vi "Write daemon error.vi"(8 "error in (no error)":errorcluster, 10 "daemon error":errorcluster, 11 "Network Slave in":refnum<class "WebSocket Server.lvclass">) -> (0 "error out":errorcluster, 3 "Network Slave out":refnum<class "WebSocket Server.lvclass">)   [LabVIEW 2021, in "WebSockets.lvlib" / "WebSocket Server.lvclass"]
uses:
  WebSocket Server.lvclass
  WebSocket Server.lvclass/WebSocket Server.ctl
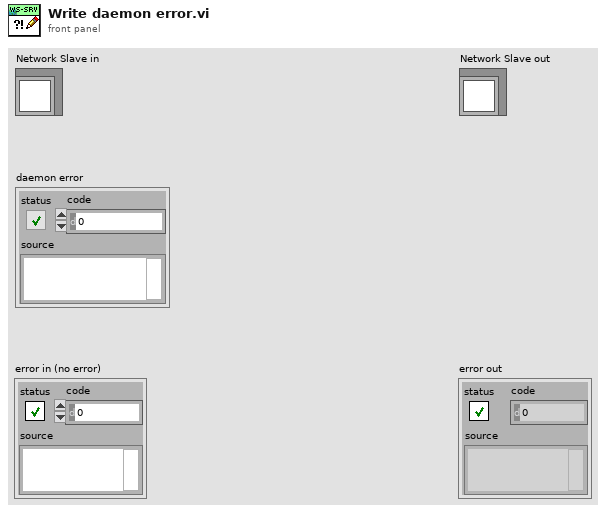
[diagram p1: front panel]
types:
  T1 = typedef "WebSockets.lvlib/WebSocket Server.lvclass/daemon status cluster.ctl" = cluster{"error":errorcluster, "status":T2}
  T2 = typedef "WebSockets.lvlib/WebSocket Server.lvclass/daemon status.ctl" = enum16{"Not Started", "Running", "Error", "Stopped"}
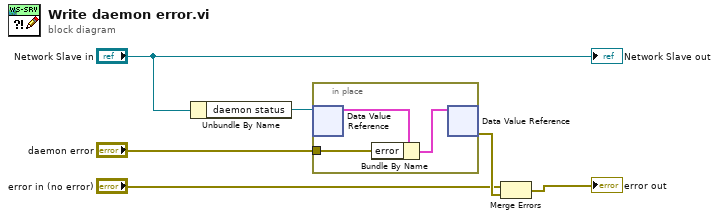
[diagram p0: block diagram]
diagram:
  n1 = Unbundle By Name("Network Slave in") -> ("daemon status"=w5:refnum<data-value>)
  n2 = in-place {
    in-place-border: "daemon error" -> [w7]
    n3 = in-place-dvr #1(w5) -> (w9:T1)  [unwired: 1 out]
    n4 = Bundle By Name(cluster=w9, "error"=w7) -> (w8:T1)
    n5 = in-place-dvr #1(w8) -> (w6:errorcluster)  [unwired: 1 out]
  }
  n6 = Merge Errors("error in (no error)", w6) -> (→"error out":errorcluster)
  "Network Slave out" <- "Network Slave in"
